vi "Create 3D Omni Wheel from Params.vi"(5 "colors":T2={"wheel color"=4884736, "roller color"=590024}, 7 "dimensions":T1={"roller thickness"=0.1, "roller radius"=0.05, "frame thickness"=0.025, "number of rollers"=6, "axle radius"=0.03, "axle length"=0.5}, 8 "error in (no error)":errorcluster, 10 "wheel radius":dbl=0.25, 11 "name":string) -> (0 "error out":errorcluster, 2 "rotation axis":refnum<vi>, 3 "3D omni wheel frame":refnum<vi>)   [LabVIEW 2017, in "NI_Robotics 3D Picture Steering Utilities.lvlib"]
doc: "Creates a 3D picture control mecanum wheel object."
uses:
  <vilib>/robotics/Steering/Utilities/3D Picture/NI_Robotics 3D Picture Steering Utilities.lvlib
  <vilib>/robotics/Steering/Utilities/3D Picture/Omni Wheel Colors.ctl
  <vilib>/robotics/Steering/Utilities/3D Picture/Omni Wheel Dimensions.ctl
  <vilib>/picture/3D Picture Control/Object/Create Object (name).vi
  <vilib>/picture/3D Picture Control/NI_3D Picture Control.lvlib
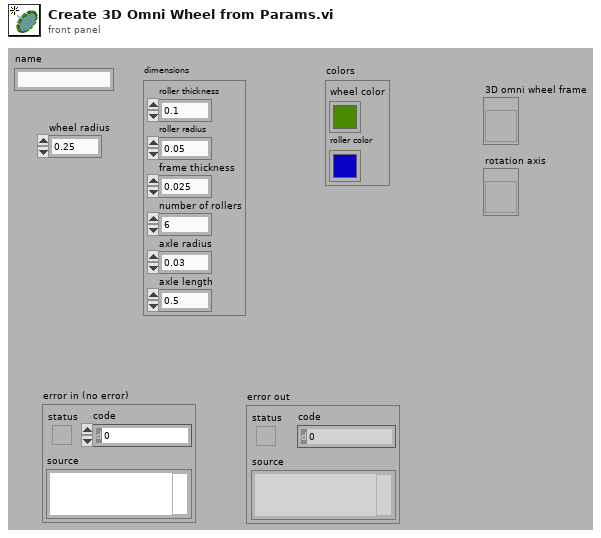
[diagram p1: front panel]
types:
  T1 = typedef "NI_Robotics 3D Picture Steering Utilities.lvlib/Omni Wheel Dimensions.ctl" = cluster{"roller thickness":dbl, "roller radius":dbl, "frame thickness":dbl, "number of rollers":i32, "axle radius":dbl, "axle length":dbl}
  T2 = typedef "NI_Robotics 3D Picture Steering Utilities.lvlib/Omni Wheel Colors.ctl" = cluster{"wheel color":u32, "roller color":u32}
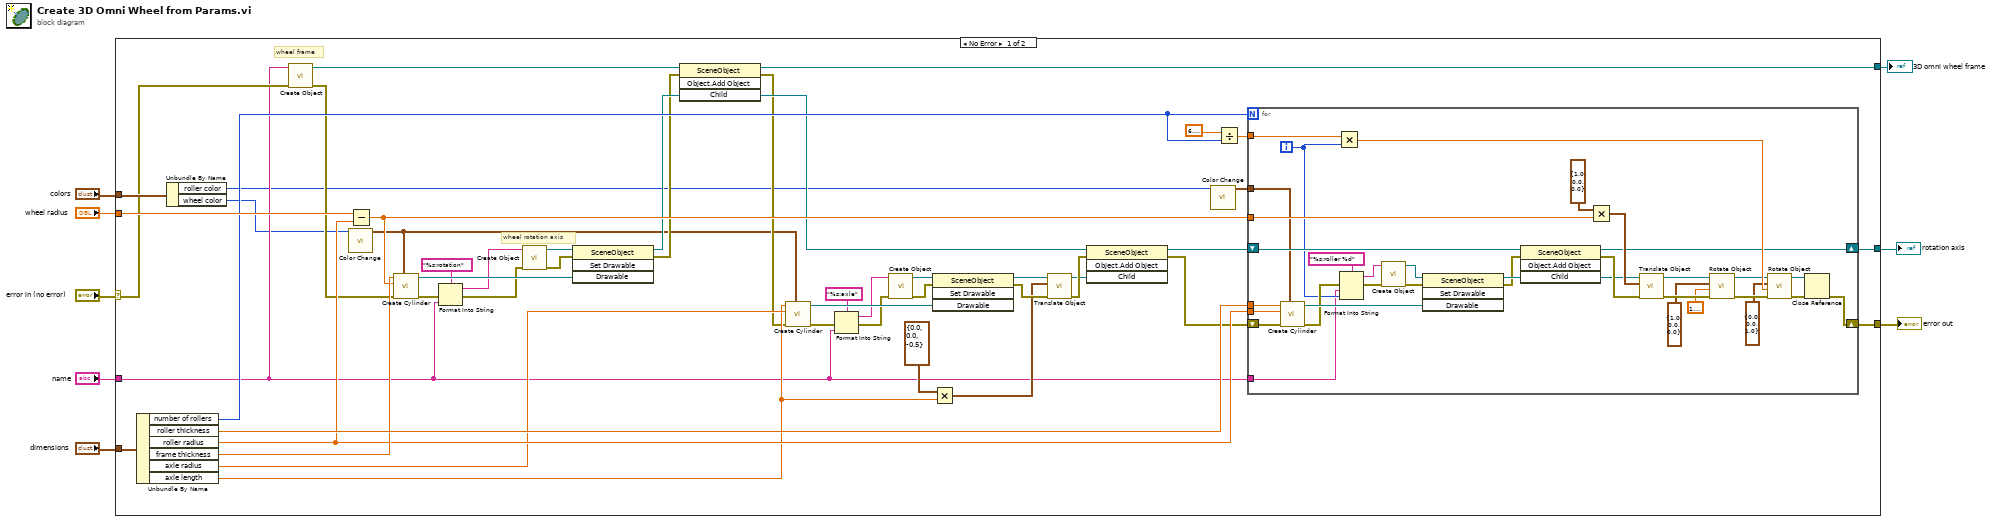
[diagram p0: block diagram]
diagram:
  n1 = case shown="No Error" "error in (no error)" {
    selector: "error in (no error)" -> [w25 w92]
    tunnel: [w55 _] -> w8
    tunnel: "dimensions" -> [w54 _]
    tunnel: "wheel radius" -> [w47 _]
    tunnel: "colors" -> [w45 _]
    tunnel: [w31 w92] -> w3
    tunnel: "name" -> [w14 _]
    tunnel: [w18 _] -> w1
    frame No Error {
      # "wheel rotation axis"
      # "wheel frame"
      n2 = Unbundle By Name(w54) -> ("number of rollers"=w26:i32, "roller thickness"=w53:dbl, "roller radius"=w48:dbl, "frame thickness"=w49:dbl, "axle radius"=w44:dbl, "axle length"=w34:dbl)
      n3 = Unbundle By Name(w45) -> ("roller color"=w10:u32, "wheel color"=w12:u32)
      n4 = call-poly <vilib>:"Create Object.vi"("error in (no error)"=w25, "Name"=w14) -> ("error out"=w24:errorcluster, "Scene:New Object"=w23:refnum<vi>)  [unwired: 8 in]
      n5 = call <vilib>:"Color Change.vi"("Color"=w12) -> ("RGBA"=w11:cluster{"R":sgl, "G":sgl, "B":sgl, "A":sgl})  [unwired: 10 in]
      n6 = Subtract(x=w47, y=w48) -> (x-y=w46:dbl)
      n7 = call <vilib>:"Create Cylinder.vi"("Color"=w11, "error in (no error)"=w24, "Radius"=w46, "Height"=w49) -> ("error out"=w17:errorcluster, "New Cylinder Refnum"=w52:refnum<vi>)  [unwired: 6 out]
      n8 = Format Into String(format string="%s:rotation", error in=w17, w14) -> (resulting string=w13:string, error out=w16:errorcluster)  [unwired: 1 in]
      n9 = call-poly <vilib>:"Create Object.vi"("error in (no error)"=w16, "Name"=w13) -> ("error out"=w50:errorcluster, "Scene:New Object"=w51:refnum<vi>)  [unwired: 8 in]
      n10 = invoke class="SceneObject" method="Set Drawable"(reference=w51, error in=w50, "Drawable"=w52) -> (reference out=w22:refnum<vi>, error out=w20:errorcluster)  [unwired: 1 in, 2 out]
      n11 = invoke class="SceneObject" method="Object.Add Object"(reference=w23, error in=w20, "Child"=w22) -> (reference out=w18:refnum<vi>, error out=w19:errorcluster, "Child"=w21:refnum<vi>)  [unwired: 1 in, 1 out]
      n12 = call <vilib>:"Create Cylinder.vi"("Color"=w11, "error in (no error)"=w19, "Radius"=w44, "Height"=w34) -> ("error out"=w30:errorcluster, "New Cylinder Refnum"=w41:refnum<vi>)  [unwired: 6 out]
      n13 = Format Into String(format string="%s:axle" ("Name"), error in=w30, w14) -> (resulting string=w27:string, error out=w29:errorcluster)  [unwired: 1 in]
      n14 = call-poly <vilib>:"Create Object.vi"("error in (no error)"=w29, "Name"=w27) -> ("error out"=w42:errorcluster, "Scene:New Object"=w43:refnum<vi>)  [unwired: 8 in]
      n15 = invoke class="SceneObject" method="Set Drawable"(reference=w43, error in=w42, "Drawable"=w41) -> (reference out=w36:refnum<vi>, error out=w38:errorcluster)  [unwired: 1 in, 2 out]
      n16 = Multiply(x=cluster{"X":sgl, "Y":sgl, "Z":sgl} {"X"=0.0, "Y"=0.0, "Z"=-0.5} ("Translation"), y=w34) -> (x*y=w32:cluster{"X":dbl, "Y":dbl, "Z":dbl})
      n17 = call <vilib>:"Translate Object.vi"("error in (no error)"=w38, "Translation"=w32, "Scene.Object In"=w36) -> ("error out"=w37:errorcluster, "Scene.Object Out"=w35:refnum<vi>)  [unwired: 7 out]
      n18 = invoke class="SceneObject" method="Object.Add Object"(reference=w21, error in=w37, "Child"=w35) -> (reference out=w40:refnum<vi>, error out=w39:errorcluster)  [unwired: 1 in, 2 out]
      n19 = call <vilib>:"Color Change.vi"("Color"=w10) -> ("RGBA"=w9:cluster{"R":sgl, "G":sgl, "B":sgl, "A":sgl})  [unwired: 10 in]
      n20 = Divide(x=6.283185307179586, y=w26) -> (x/y=w56:dbl)
      n21 = for {
        N: w26 -> [_]
        tunnel: w48 -> [w91]
        tunnel: w46 -> [w82]
        tunnel: w56 -> [w85]
        shift-right: [w65] -> w31
        shift-left: w39 -> [w80]
        shift-right: [w64] -> w55
        shift-left: w40 -> [w67]
        tunnel: w53 -> [w63]
        tunnel: w9 -> [w62]
        tunnel: w14 -> [w60]
        i -> [w61]
        n22 = call <vilib>:"Create Cylinder.vi"("Color"=w62, "error in (no error)"=w80, "Radius"=w91, "Height"=w63) -> ("error out"=w79:errorcluster, "New Cylinder Refnum"=w86:refnum<vi>)  [unwired: 6 out]
        n23 = Multiply(x=w85, y=w61) -> (x*y=w84:dbl)
        n24 = Format Into String(format string="%s:roller %d", error in=w79, w60, w61) -> (resulting string=w68:string, error out=w89:errorcluster)  [unwired: 1 in]
        n25 = call-poly <vilib>:"Create Object.vi"("error in (no error)"=w89, "Name"=w68) -> ("error out"=w88:errorcluster, "Scene:New Object"=w87:refnum<vi>)  [unwired: 8 in]
        n26 = invoke class="SceneObject" method="Set Drawable"(reference=w87, error in=w88, "Drawable"=w86) -> (reference out=w78:refnum<vi>, error out=w66:errorcluster)  [unwired: 1 in, 2 out]
        n27 = invoke class="SceneObject" method="Object.Add Object"(reference=w67, error in=w66, "Child"=w78) -> (reference out=w64:refnum<vi>, error out=w77:errorcluster, "Child"=w76:refnum<vi>)  [unwired: 1 in, 1 out]
        n28 = Multiply(x=cluster{"X":sgl, "Y":sgl, "Z":sgl} {"X"=1.0, "Y"=0.0, "Z"=0.0} ("Translation"), y=w82) -> (x*y=w81:cluster{"X":dbl, "Y":dbl, "Z":dbl})
        n29 = call <vilib>:"Translate Object.vi"("error in (no error)"=w77, "Translation"=w81, "Scene.Object In"=w76) -> ("error out"=w75:errorcluster, "Scene.Object Out"=w74:refnum<vi>)  [unwired: 7 out]
        n30 = call <vilib>:"Rotate Object.vi"("error in (no error)"=w75, "Angle"=1.5707963267948966, "Axis"=cluster{"X":sgl, "Y":sgl, "Z":sgl} {"X"=1.0, "Y"=0.0, "Z"=0.0}, "Scene.Object In"=w74) -> ("error out"=w73:errorcluster, "Scene.Object Out"=w72:refnum<vi>)  [unwired: 6 out]
        n31 = call <vilib>:"Rotate Object.vi"("error in (no error)"=w73, "Angle"=w84, "Axis"=cluster{"X":sgl, "Y":sgl, "Z":sgl} {"X"=0.0, "Y"=0.0, "Z"=1.0}, "Scene.Object In"=w72) -> ("error out"=w70:errorcluster, "Scene.Object Out"=w71:refnum<vi>)  [unwired: 6 out]
        n32 = Close Reference(reference=w71, error in (no error)=w70) -> (error out=w65:errorcluster)
      }
    }
    frame Error {
    }
  }
  "rotation axis" <- w8
  "error out" <- w3
  "3D omni wheel frame" <- w1
